vi "oa_Extract Even Angle Signal by Indice(N CH).vi"(0 "even angle signals":cluster{"r0":dbl, "dr":dbl, "Y":dbl[]}[](array[cluster]) {"r0" format="%.2p"; "dr" format="%.2p"; "Y" format="%.2f"}, 1 "reset?":bool, 7 "trigger indices":T1, 11 "block size":i32=1024 min=2, 12 "indices end?":bool) -> (3 "new signal available?":bool, 4 "even angle signals output":cluster{"r0":dbl, "dr":dbl, "Y":dbl[]}[](array[cluster]), 14 "reached end?":bool, 15 "current position":cluster{"rev":dbl, "time":dbl, "RPM":dbl})   [LabVIEW 2017, in "SoundVib_OAUtility.lvlib"]
uses:
  <vilib>/addons/Sound and Vibration/Order Analysis/Utility/SoundVib_OAUtility.lvlib
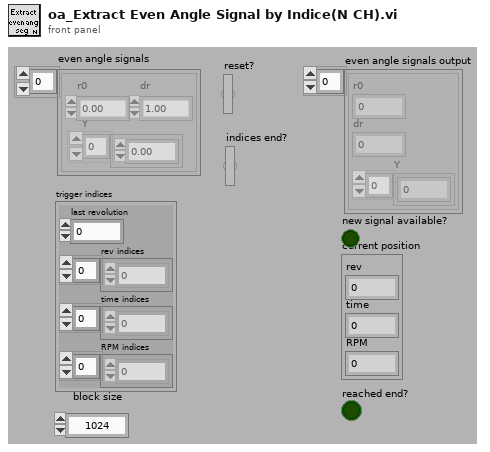
[diagram p1: front panel]
types:
  T1 = cluster{"last revolution":dbl, "rev indices":dbl[], "time indices":dbl[], "RPM indices":dbl[]}
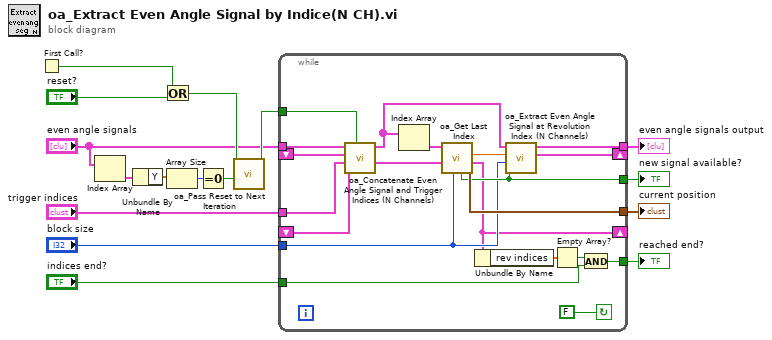
[diagram p0: block diagram]
diagram:
  n1 = First Call?() -> (First Call?: T/F=w11:bool)
  n2 = Index Array(array="even angle signals") -> (element=w16:cluster{"r0":dbl, "dr":dbl, "Y":dbl[]})  [unwired: 1 in]
  n3 = Unbundle By Name(w16) -> ("Y"=w15:dbl[])
  n4 = Or(x=w11, y="reset?") -> (x .or. y?=w9:bool)
  n5 = Array Size(array=w15) -> (size(s)=w14:i32)
  n6 = Equal To 0?(x=w14) -> (x = 0?=w10:bool)
  n7 = call <vilib>:"oa_Pass Reset to Next Iteration.vi"("trigger"=w10, "reset?(F)"=w9) -> ("reset out"=w13:bool)  [unwired: 9 in]
  n8 = while {
    tunnel: w13 -> [w31]
    shift-right: [w26] -> _
    shift-left: _ -> [w33]
    tunnel: "even angle signals" -> [w32]
    tunnel: "block size" -> [w22]
    tunnel: "trigger indices" -> [w34]
    shift-right: [w21] -> _
    shift-left: _ -> [w35]
    tunnel: [w29] -> w4
    tunnel: [w27] -> w5
    tunnel: [w23] -> w3
    tunnel: "indices end?" -> [w18]
    tunnel: [w17] -> w1
    stop <- FALSE continue-if-true
    n9 = call <vilib>:"oa_Concatenate Even Angle Signal and Trigger Indices (N Channels).vi"("reset?"=w31, "history trigger indices"=w35, "trigger indices"=w34, "history even angle signals"=w33, "even angle signals"=w32) -> ("trigger indices out"=w30:T1, "even angle signals out"=w24:cluster{"r0":dbl, "dr":dbl, "Y":dbl[]}[])  [unwired: 5 in]
    n10 = Index Array(array=w24) -> (element=w25:cluster{"r0":dbl, "dr":dbl, "Y":dbl[]})  [unwired: 1 in]
    n11 = call <vilib>:"oa_Get Last Index.vi"("block size"=w22, "trigger indices"=w30, "even angle signal"=w25) -> ("current positon"=w29:cluster{"rev":dbl, "time":dbl, "RPM":dbl}, "trigger indices for buffer"=w21:T1, "rev index"=w28:dbl, "index in range"=w23:bool)  [unwired: 5 in]
    n12 = Unbundle By Name(w21) -> ("rev indices"=w20:dbl[])
    n13 = call <vilib>:"oa_Extract Even Angle Signal at Revolution Index (N Channels).vi"("index in range"=w23, "block size"=w22, "rev index"=w28, "even angle signals"=w24) -> ("even angle signals for buffer"=w26:cluster{"r0":dbl, "dr":dbl, "Y":dbl[]}[], "even angle signals out"=w27:cluster{"r0":dbl, "dr":dbl, "Y":dbl[]}[])  [unwired: 6 in]
    n14 = Empty Array?(array=w20) -> (empty?=w19:bool)
    n15 = And(x=w19, y=w18) -> (x .and. y?=w17:bool)
  }
  "even angle signals output" <- w5
  "current position" <- w4
  "new signal available?" <- w3
  "reached end?" <- w1
